vi "Update_usb_names.vi"(10 "Friendly Name ref":refnum<vi>, 11 "Serial Devices ref":refnum<vi>) -> ()   [LabVIEW 2012]
uses:
  <vilib>/Instr/_visa.llb/VISA Find Search Mode.ctl
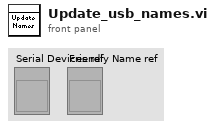
[diagram p1: front panel]
types:
  T1 = typedef "VISA Find Search Mode.ctl" = u32
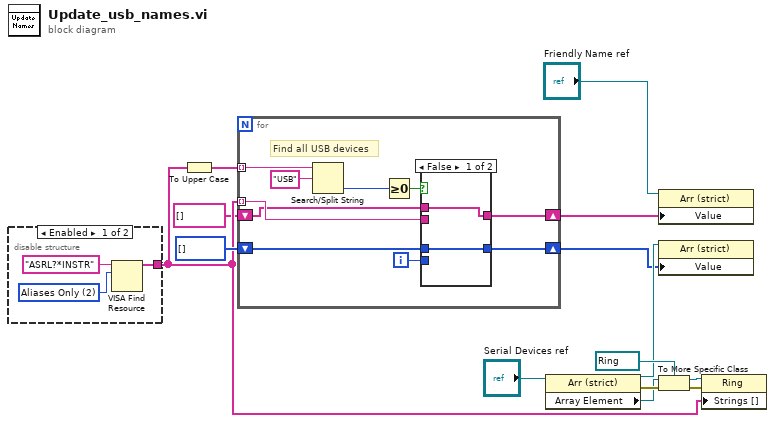
[diagram p0: block diagram]
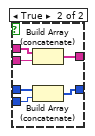
[diagram p2: hidden frame]
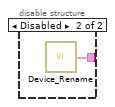
[diagram p3: hidden frame]
diagram:
  n1 = disable-structure shown="Enabled" {
    disable-tunnel: [w15 w18] -> w3
    frame Enabled {
      w17 = T1 2 items=["Canonical Names Only"=0, "Aliases Only"=2, "Include Matching Aliases"=3, "Include All Aliases"=4] ("Search Mode")
      n2 = VISA Find Resource(10:w17, 11:"ASRL?*INSTR" ("expression (\"?*\")")) -> (3:w15:string[])  [unwired: 1 in, 2 out]
    }
    frame Disabled {
      n3 = call "Device_Rename.vi"() -> ("Aliases"=w18:string[])  [unwired: 3 in, 2 out]
    }
  }
  n4 = To Upper Case(1:w3) -> (0:w8:string[])
  n5 = for {
    tunnel: w8 -> [w26] mode=indexing
    shift-right: [w23] -> w5
    shift-left: i32[] [] -> [w22]
    tunnel: w3 -> [w21] mode=indexing
    shift-right: [w20] -> w1
    shift-left: string[] [] -> [w19]
    i -> [w24]
    # "Find all USB devices"
    n6 = Search/Split String(string=w26, search string/char (-)="USB") -> (offset of match=w27:i32)  [unwired: 1 in, 2 out]
    n7 = Greater Or Equal To 0?(x=w27) -> (x >= 0?=w25:bool)
    n8 = case shown="False" w25 {
      tunnel: w24 -> [_ w36]
      tunnel: [w30 w35] -> w23
      tunnel: w22 -> [w30 w34]
      tunnel: w21 -> [_ w33]
      tunnel: [w29 w32] -> w20
      tunnel: w19 -> [w29 w31]
      frame False {
      }
      frame True {
        n9 = Build Array (concatenate)(w31, w33) -> (w32:string[])
        n10 = Build Array (concatenate)(w34, w36) -> (w35:i32[])
      }
    }
  }
  n11 = property class="Arr (strict)"(reference="Serial Devices ref") -> (reference out=w6:refnum<vi>, error out=w11:errorcluster, "Array Element"=w10:refnum<vi>)  [unwired: 1 in]
  n12 = property class="Arr (strict)"(reference="Friendly Name ref", "Value"=w1) -> ()  [unwired: 1 in, 2 out]
  n13 = property class="Arr (strict)"(reference=w6, "Value"=w5) -> ()  [unwired: 1 in, 2 out]
  n14 = To More Specific Class(target class=refnum<vi> refnum ("Protocols"), reference=w10, error in=w11) -> (specific class reference=w13:refnum<vi>, error out=w14:errorcluster)
  n15 = property class="Ring"(reference=w13, error in=w14, "Strings []"=w3) -> ()  [unwired: 2 out]
